vi "rethinkdb_json_type_cast.vi"(7 "type":variant, 8 "error in (no error)":errorcluster, 9 "allow missing? (F)":bool, 11 "json object":variant) -> (0 "error out":errorcluster, 1 "all keys found?":bool, 2 "data string":string, 3 "type string":i16[](array[numeric]))   [LabVIEW 2017]
uses:
  <vilib>/Utility/Data Type/Type Definitions/Data Type.ctl
  <vilib>/Utility/Data Type/NI_Data Type.lvlib
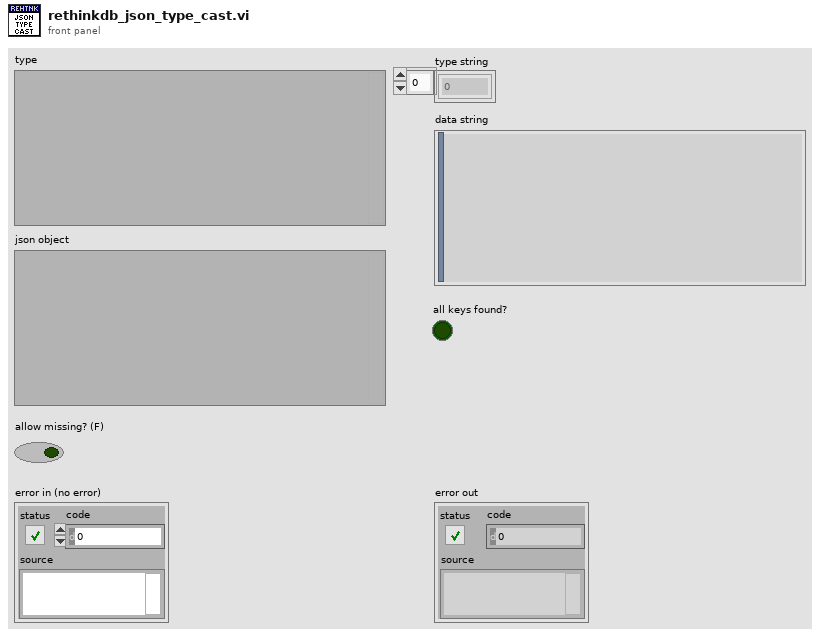
[diagram p1: front panel]
types:
  T1 = typedef "NI_Data Type.lvlib/Data Type.ctl" = enum8{"Invalid Type", "Void", "I8", "I16", "I32", "I64", "U8", "U16", "U32", "U64", "Single Float", "Double Float", "Extended Float", "Single Complex", "Double Complex", "Extended Complex", "Enum U8", "Enum U16", "Enum U32", "Enum U64", "Single Float With Unit", "Double Float With Unit", "Extended Float With Unit", "Single Complex with Unit", "Double Complex with Unit", "Extended Complex with Unit", "Boolean", "String", "Path", "Picture", "Tag", "Array", "Cluster", "Variant", "LV Variant", "Waveform", "Timestamp", "Digital Waveform", "Digital Data", "ExpressData", "Refnum", "External Data", "VI", "Poly VI", "LabVIEW Class Instance", "Fixed Point"}
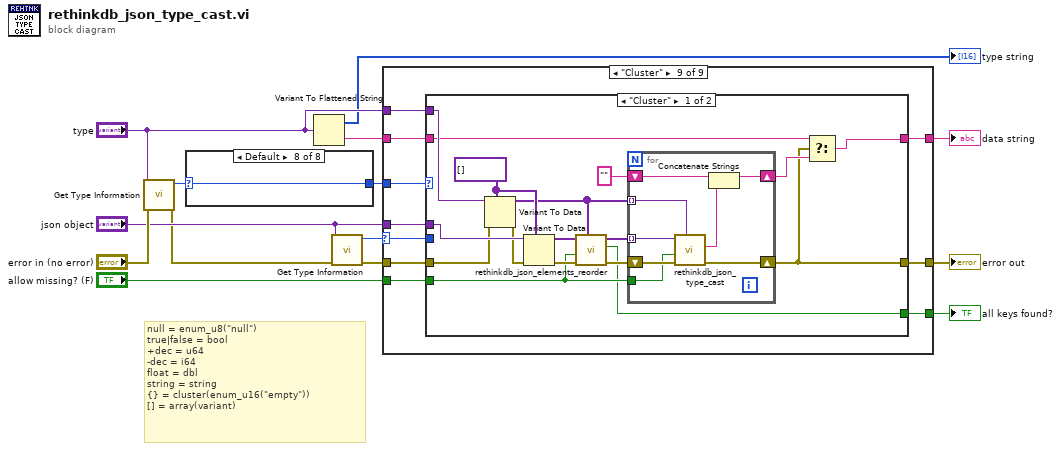
[diagram p0: block diagram]
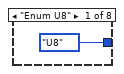
[diagram p2: hidden frame]
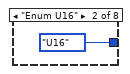
[diagram p3: hidden frame]
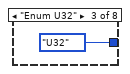
[diagram p4: hidden frame]
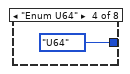
[diagram p5: hidden frame]
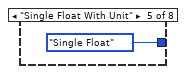
[diagram p6: hidden frame]
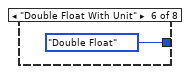
[diagram p7: hidden frame]
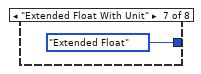
[diagram p8: hidden frame]
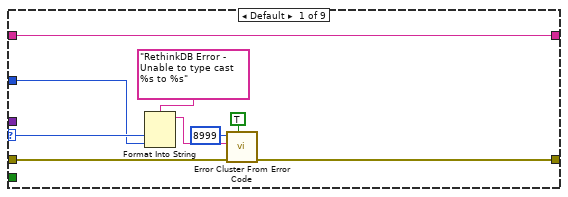
[diagram p9: hidden frame]
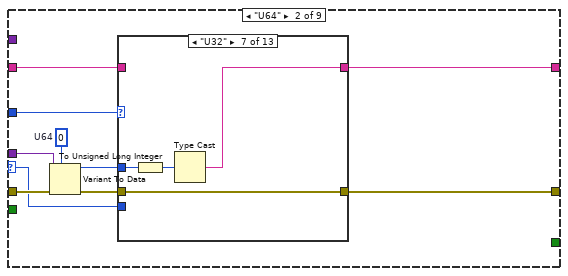
[diagram p10: hidden frame]
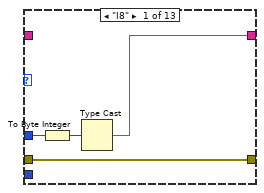
[diagram p11: hidden frame]
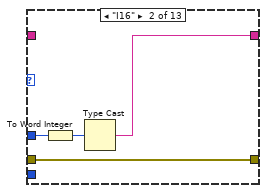
[diagram p12: hidden frame]
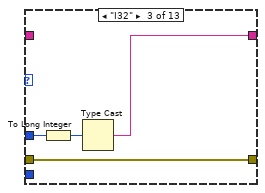
[diagram p13: hidden frame]
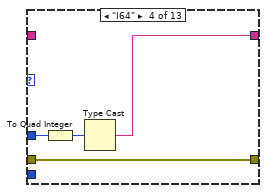
[diagram p14: hidden frame]
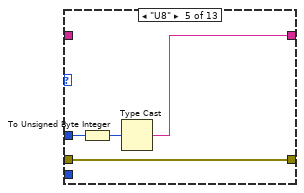
[diagram p15: hidden frame]
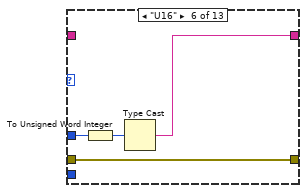
[diagram p16: hidden frame]
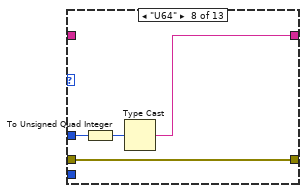
[diagram p17: hidden frame]
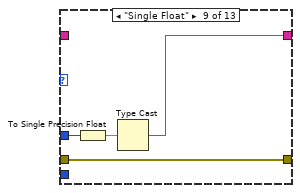
[diagram p18: hidden frame]
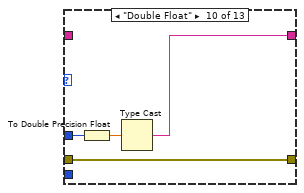
[diagram p19: hidden frame]
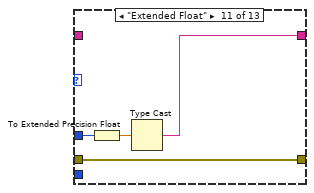
[diagram p20: hidden frame]
diagram:
  # "null = enum_u8(\"null\")\ntrue|false = bool\n+dec = u64\n-dec = i64\nfloat = dbl\nstring = string\n{} = cluster(enum_u16(\"empty\"))\n[] = array(variant)"
  n1 = call <vilib>:"Get Type Information.vi"("error in (no error)"="error in (no error)", "Variant"="type") -> ("error out"=w9:errorcluster, "Type"=w6:T1)  [unwired: 5 in, 3 out]
  n2 = case shown="Default" w6 {
    selector: w6 -> [_ _ _ _ _ _ _ w22]
    tunnel: [Data_Type."U8" ("Type") Data_Type."U16" ("Type") Data_Type."U32" ("Type") Data_Type."U64" ("Type") Data_Type."Single Float" ("Type") Data_Type."Double Float" ("Type") Data_Type."Extended Float" ("Type") w22] -> w5
    frame "Enum U8" {
    }
    frame "Enum U16" {
    }
    frame "Enum U32" {
    }
    frame "Enum U64" {
    }
    frame "Single Float With Unit" {
    }
    frame "Double Float With Unit" {
    }
    frame "Extended Float With Unit" {
    }
    frame Default {
    }
  }
  n3 = Variant To Flattened String(Variant="type") -> (data string=w4:string, 1:→"type string":i16[])
  n4 = call <vilib>:"Get Type Information.vi"("error in (no error)"=w9, "Variant"="json object") -> ("error out"=w7:errorcluster, "Type"=w8:T1)  [unwired: 5 in, 3 out]
  n5 = case shown="\"Cluster\"" w8 {
    selector: w8 -> [w25 w34 w102 w169 w235 w303 _ _ w368]
    tunnel: w7 -> [w31 w41 w108 w175 w243 w310 w332 w351 w367]
    tunnel: [w30 w35 w99 w166 w236 w304 w327 w346 w370] -> w12
    tunnel: w5 -> [w24 w37 w104 w171 w240 w307 w329 w348 w369]
    tunnel: "json object" -> [_ w40 w107 w174 w242 w309 w331 w350 w366]
    tunnel: w4 -> [w23 w33 w101 w168 w234 w302 w325 w344 w364]
    tunnel: [w23 w32 w100 w167 w233 w301 w324 w344 w365] -> w10
    tunnel: "type" -> [_ _ _ _ _ _ _ _ w363]
    tunnel: "allow missing? (F)" -> [_ _ _ _ _ _ _ _ w362]
    tunnel: [_ _ _ _ _ _ _ _ w361] -> w1
    frame Default {
      n6 = Format Into String(format string="RethinkDB Error - Unable to type cast %s to %s" ("error message (\"\")"), w25, w24) -> (resulting string=w26:string)  [unwired: 2 in, 1 out]
      n7 = call <vilib>:"Error Cluster From Error Code.vi"("show call chain? (False)"=TRUE, "error in (no error)"=w31, "error message (\"\")"=w26, "error code (0)"=8999) -> ("error out"=w30:errorcluster)  [unwired: 5 in]
    }
    frame "U64" {
      w39 = u64 0  # U64
      n8 = Variant To Data(error in=w41, type=w39, Variant=w40) -> (data=w36:u64, error out=w38:errorcluster)
      n9 = case shown="\"U32\"" w37 {
        selector: w37 -> [_ _ _ _ _ _ _ _ _ _ _ _ w91]
        tunnel: [w45 w49 w53 w57 w61 w65 w69 w73 w77 w81 w85 w89 w92] -> w35
        tunnel: w38 -> [w45 w49 w53 w57 w61 w65 w69 w73 w77 w81 w85 w89 w93]
        tunnel: w36 -> [w44 w48 w52 w56 w60 w64 w68 w72 w76 w80 w84 w87 _]
        tunnel: [w42 w46 w50 w54 w58 w62 w66 w70 w74 w78 w82 w88 w98] -> w32
        tunnel: w33 -> [_ _ _ _ _ _ _ _ _ _ _ _ w98]
        tunnel: w34 -> [_ _ _ _ _ _ _ _ _ _ _ _ w90]
        frame "I8" {
          n10 = To Byte Integer(number=w44) -> (8bit integer=w43:i8)
          n11 = Type Cast(x=w43) -> (*(type *) &x=w42:string)  [unwired: 1 in]
        }
        frame "I16" {
          n12 = To Word Integer(number=w48) -> (16bit integer=w47:i16)
          n13 = Type Cast(x=w47) -> (*(type *) &x=w46:string)  [unwired: 1 in]
        }
        frame "I32" {
          n14 = To Long Integer(number=w52) -> (32bit integer=w51:i32)
          n15 = Type Cast(x=w51) -> (*(type *) &x=w50:string)  [unwired: 1 in]
        }
        frame "I64" {
          n16 = To Quad Integer(1:w56) -> (0:w55:i64)
          n17 = Type Cast(x=w55) -> (*(type *) &x=w54:string)  [unwired: 1 in]
        }
        frame "U8" {
          n18 = To Unsigned Byte Integer(number=w60) -> (unsigned 8bit integer=w59:u8)
          n19 = Type Cast(x=w59) -> (*(type *) &x=w58:string)  [unwired: 1 in]
        }
        frame "U16" {
          n20 = To Unsigned Word Integer(number=w64) -> (unsigned 16bit integer=w63:u16)
          n21 = Type Cast(x=w63) -> (*(type *) &x=w62:string)  [unwired: 1 in]
        }
        frame "U32" {
          n22 = To Unsigned Long Integer(number=w68) -> (unsigned 32bit integer=w67:u32)
          n23 = Type Cast(x=w67) -> (*(type *) &x=w66:string)  [unwired: 1 in]
        }
        frame "U64" {
          n24 = To Unsigned Quad Integer(1:w72) -> (0:w71:u64)
          n25 = Type Cast(x=w71) -> (*(type *) &x=w70:string)  [unwired: 1 in]
        }
        frame "Single Float" {
          n26 = To Single Precision Float(number=w76) -> (single precision float=w75:sgl)
          n27 = Type Cast(x=w75) -> (*(type *) &x=w74:string)  [unwired: 1 in]
        }
        frame "Double Float" {
          n28 = To Double Precision Float(number=w80) -> (double precision float=w79:dbl)
          n29 = Type Cast(x=w79) -> (*(type *) &x=w78:string)  [unwired: 1 in]
        }
        frame "Extended Float" {
          n30 = To Extended Precision Float(1:w84) -> (0:w83:ext)
          n31 = Type Cast(x=w83) -> (*(type *) &x=w82:string)  [unwired: 1 in]
        }
        frame "Boolean" {
          n32 = Not Equal To 0?(x=w87) -> (x != 0?=w86:bool)
          n33 = Type Cast(x=w86) -> (*(type *) &x=w88:string)  [unwired: 1 in]
        }
        frame Default {
          n34 = Format Into String(format string="RethinkDB Error - Unable to type cast %s to %s" ("error message (\"\")"), w90, w91) -> (resulting string=w94:string)  [unwired: 2 in, 1 out]
          n35 = call <vilib>:"Error Cluster From Error Code.vi"("show call chain? (False)"=TRUE, "error in (no error)"=w93, "error message (\"\")"=w94, "error code (0)"=8999) -> ("error out"=w92:errorcluster)  [unwired: 5 in]
        }
      }
    }
    frame "I64" {
      w106 = i64 0  # I64
      n36 = Variant To Data(error in=w108, type=w106, Variant=w107) -> (data=w103:i64, error out=w105:errorcluster)
      n37 = case shown="Default" w104 {
        selector: w104 -> [_ _ _ _ _ _ _ _ _ _ _ _ w158]
        tunnel: [w112 w116 w120 w124 w128 w132 w136 w140 w144 w148 w152 w156 w159] -> w99
        tunnel: w105 -> [w112 w116 w120 w124 w128 w132 w136 w140 w144 w148 w152 w156 w160]
        tunnel: w103 -> [w111 w115 w119 w123 w127 w131 w135 w139 w143 w147 w151 w154 _]
        tunnel: [w109 w113 w117 w121 w125 w129 w133 w137 w141 w145 w149 w155 w165] -> w100
        tunnel: w101 -> [_ _ _ _ _ _ _ _ _ _ _ _ w165]
        tunnel: w102 -> [_ _ _ _ _ _ _ _ _ _ _ _ w157]
        frame "I8" {
          n38 = To Byte Integer(number=w111) -> (8bit integer=w110:i8)
          n39 = Type Cast(x=w110) -> (*(type *) &x=w109:string)  [unwired: 1 in]
        }
        frame "I16" {
          n40 = To Word Integer(number=w115) -> (16bit integer=w114:i16)
          n41 = Type Cast(x=w114) -> (*(type *) &x=w113:string)  [unwired: 1 in]
        }
        frame "I32" {
          n42 = To Long Integer(number=w119) -> (32bit integer=w118:i32)
          n43 = Type Cast(x=w118) -> (*(type *) &x=w117:string)  [unwired: 1 in]
        }
        frame "I64" {
          n44 = To Quad Integer(1:w123) -> (0:w122:i64)
          n45 = Type Cast(x=w122) -> (*(type *) &x=w121:string)  [unwired: 1 in]
        }
        frame "U8" {
          n46 = To Unsigned Byte Integer(number=w127) -> (unsigned 8bit integer=w126:u8)
          n47 = Type Cast(x=w126) -> (*(type *) &x=w125:string)  [unwired: 1 in]
        }
        frame "U16" {
          n48 = To Unsigned Word Integer(number=w131) -> (unsigned 16bit integer=w130:u16)
          n49 = Type Cast(x=w130) -> (*(type *) &x=w129:string)  [unwired: 1 in]
        }
        frame "U32" {
          n50 = To Unsigned Long Integer(number=w135) -> (unsigned 32bit integer=w134:u32)
          n51 = Type Cast(x=w134) -> (*(type *) &x=w133:string)  [unwired: 1 in]
        }
        frame "U64" {
          n52 = To Unsigned Quad Integer(1:w139) -> (0:w138:u64)
          n53 = Type Cast(x=w138) -> (*(type *) &x=w137:string)  [unwired: 1 in]
        }
        frame "Single Float" {
          n54 = To Single Precision Float(number=w143) -> (single precision float=w142:sgl)
          n55 = Type Cast(x=w142) -> (*(type *) &x=w141:string)  [unwired: 1 in]
        }
        frame "Double Float" {
          n56 = To Double Precision Float(number=w147) -> (double precision float=w146:dbl)
          n57 = Type Cast(x=w146) -> (*(type *) &x=w145:string)  [unwired: 1 in]
        }
        frame "Extended Float" {
          n58 = To Extended Precision Float(1:w151) -> (0:w150:ext)
          n59 = Type Cast(x=w150) -> (*(type *) &x=w149:string)  [unwired: 1 in]
        }
        frame "Boolean" {
          n60 = Not Equal To 0?(x=w154) -> (x != 0?=w153:bool)
          n61 = Type Cast(x=w153) -> (*(type *) &x=w155:string)  [unwired: 1 in]
        }
        frame Default {
          n62 = Format Into String(format string="RethinkDB Error - Unable to type cast %s to %s" ("error message (\"\")"), w157, w158) -> (resulting string=w161:string)  [unwired: 2 in, 1 out]
          n63 = call <vilib>:"Error Cluster From Error Code.vi"("show call chain? (False)"=TRUE, "error in (no error)"=w160, "error message (\"\")"=w161, "error code (0)"=8999) -> ("error out"=w159:errorcluster)  [unwired: 5 in]
        }
      }
    }
    frame "Double Float" {
      w173 = 0.0  # DBL
      n64 = Variant To Data(error in=w175, type=w173, Variant=w174) -> (data=w170:dbl, error out=w172:errorcluster)
      n65 = case shown="Default" w171 {
        selector: w171 -> [_ _ _ _ _ _ _ _ _ _ _ _ w225]
        tunnel: [w179 w183 w187 w191 w195 w199 w203 w207 w211 w215 w219 w223 w226] -> w166
        tunnel: w172 -> [w179 w183 w187 w191 w195 w199 w203 w207 w211 w215 w219 w223 w227]
        tunnel: w170 -> [w178 w182 w186 w190 w194 w198 w202 w206 w210 w214 w218 w221 _]
        tunnel: [w176 w180 w184 w188 w192 w196 w200 w204 w208 w212 w216 w222 w232] -> w167
        tunnel: w168 -> [_ _ _ _ _ _ _ _ _ _ _ _ w232]
        tunnel: w169 -> [_ _ _ _ _ _ _ _ _ _ _ _ w224]
        frame "I8" {
          n66 = To Byte Integer(number=w178) -> (8bit integer=w177:i8)
          n67 = Type Cast(x=w177) -> (*(type *) &x=w176:string)  [unwired: 1 in]
        }
        frame "I16" {
          n68 = To Word Integer(number=w182) -> (16bit integer=w181:i16)
          n69 = Type Cast(x=w181) -> (*(type *) &x=w180:string)  [unwired: 1 in]
        }
        frame "I32" {
          n70 = To Long Integer(number=w186) -> (32bit integer=w185:i32)
          n71 = Type Cast(x=w185) -> (*(type *) &x=w184:string)  [unwired: 1 in]
        }
        frame "I64" {
          n72 = To Quad Integer(1:w190) -> (0:w189:i64)
          n73 = Type Cast(x=w189) -> (*(type *) &x=w188:string)  [unwired: 1 in]
        }
        frame "U8" {
          n74 = To Unsigned Byte Integer(number=w194) -> (unsigned 8bit integer=w193:u8)
          n75 = Type Cast(x=w193) -> (*(type *) &x=w192:string)  [unwired: 1 in]
        }
        frame "U16" {
          n76 = To Unsigned Word Integer(number=w198) -> (unsigned 16bit integer=w197:u16)
          n77 = Type Cast(x=w197) -> (*(type *) &x=w196:string)  [unwired: 1 in]
        }
        frame "U32" {
          n78 = To Unsigned Long Integer(number=w202) -> (unsigned 32bit integer=w201:u32)
          n79 = Type Cast(x=w201) -> (*(type *) &x=w200:string)  [unwired: 1 in]
        }
        frame "U64" {
          n80 = To Unsigned Quad Integer(1:w206) -> (0:w205:u64)
          n81 = Type Cast(x=w205) -> (*(type *) &x=w204:string)  [unwired: 1 in]
        }
        frame "Single Float" {
          n82 = To Single Precision Float(number=w210) -> (single precision float=w209:sgl)
          n83 = Type Cast(x=w209) -> (*(type *) &x=w208:string)  [unwired: 1 in]
        }
        frame "Double Float" {
          n84 = To Double Precision Float(number=w214) -> (double precision float=w213:dbl)
          n85 = Type Cast(x=w213) -> (*(type *) &x=w212:string)  [unwired: 1 in]
        }
        frame "Extended Float" {
          n86 = To Extended Precision Float(1:w218) -> (0:w217:ext)
          n87 = Type Cast(x=w217) -> (*(type *) &x=w216:string)  [unwired: 1 in]
        }
        frame "Boolean" {
          n88 = Not Equal To 0?(x=w221) -> (x != 0?=w220:bool)
          n89 = Type Cast(x=w220) -> (*(type *) &x=w222:string)  [unwired: 1 in]
        }
        frame Default {
          n90 = Format Into String(format string="RethinkDB Error - Unable to type cast %s to %s" ("error message (\"\")"), w224, w225) -> (resulting string=w228:string)  [unwired: 2 in, 1 out]
          n91 = call <vilib>:"Error Cluster From Error Code.vi"("show call chain? (False)"=TRUE, "error in (no error)"=w227, "error message (\"\")"=w228, "error code (0)"=8999) -> ("error out"=w226:errorcluster)  [unwired: 5 in]
        }
      }
    }
    frame "Boolean" {
      n92 = Variant To Data(error in=w243, type=FALSE, Variant=w242) -> (data=w239:bool, error out=w241:errorcluster)
      n93 = Boolean To (0,1)(Boolean=w239) -> (0, 1=w237:i16)
      n94 = case shown="Default" w240 {
        selector: w240 -> [_ _ _ _ _ _ _ _ _ _ _ _ w293]
        tunnel: [w247 w251 w255 w259 w263 w267 w271 w275 w279 w283 w287 w291 w294] -> w236
        tunnel: w241 -> [w247 w251 w255 w259 w263 w267 w271 w275 w279 w283 w287 w291 w295]
        tunnel: w237 -> [w246 w250 w254 w258 w262 w266 w270 w274 w278 w282 w286 w289 _]
        tunnel: [w244 w248 w252 w256 w260 w264 w268 w272 w276 w280 w284 w290 w300] -> w233
        tunnel: w234 -> [_ _ _ _ _ _ _ _ _ _ _ _ w300]
        tunnel: w235 -> [_ _ _ _ _ _ _ _ _ _ _ _ w292]
        frame "I8" {
          n95 = To Byte Integer(number=w246) -> (8bit integer=w245:i8)
          n96 = Type Cast(x=w245) -> (*(type *) &x=w244:string)  [unwired: 1 in]
        }
        frame "I16" {
          n97 = To Word Integer(number=w250) -> (16bit integer=w249:i16)
          n98 = Type Cast(x=w249) -> (*(type *) &x=w248:string)  [unwired: 1 in]
        }
        frame "I32" {
          n99 = To Long Integer(number=w254) -> (32bit integer=w253:i32)
          n100 = Type Cast(x=w253) -> (*(type *) &x=w252:string)  [unwired: 1 in]
        }
        frame "I64" {
          n101 = To Quad Integer(1:w258) -> (0:w257:i64)
          n102 = Type Cast(x=w257) -> (*(type *) &x=w256:string)  [unwired: 1 in]
        }
        frame "U8" {
          n103 = To Unsigned Byte Integer(number=w262) -> (unsigned 8bit integer=w261:u8)
          n104 = Type Cast(x=w261) -> (*(type *) &x=w260:string)  [unwired: 1 in]
        }
        frame "U16" {
          n105 = To Unsigned Word Integer(number=w266) -> (unsigned 16bit integer=w265:u16)
          n106 = Type Cast(x=w265) -> (*(type *) &x=w264:string)  [unwired: 1 in]
        }
        frame "U32" {
          n107 = To Unsigned Long Integer(number=w270) -> (unsigned 32bit integer=w269:u32)
          n108 = Type Cast(x=w269) -> (*(type *) &x=w268:string)  [unwired: 1 in]
        }
        frame "U64" {
          n109 = To Unsigned Quad Integer(1:w274) -> (0:w273:u64)
          n110 = Type Cast(x=w273) -> (*(type *) &x=w272:string)  [unwired: 1 in]
        }
        frame "Single Float" {
          n111 = To Single Precision Float(number=w278) -> (single precision float=w277:sgl)
          n112 = Type Cast(x=w277) -> (*(type *) &x=w276:string)  [unwired: 1 in]
        }
        frame "Double Float" {
          n113 = To Double Precision Float(number=w282) -> (double precision float=w281:dbl)
          n114 = Type Cast(x=w281) -> (*(type *) &x=w280:string)  [unwired: 1 in]
        }
        frame "Extended Float" {
          n115 = To Extended Precision Float(1:w286) -> (0:w285:ext)
          n116 = Type Cast(x=w285) -> (*(type *) &x=w284:string)  [unwired: 1 in]
        }
        frame "Boolean" {
          n117 = Not Equal To 0?(x=w289) -> (x != 0?=w288:bool)
          n118 = Type Cast(x=w288) -> (*(type *) &x=w290:string)  [unwired: 1 in]
        }
        frame Default {
          n119 = Format Into String(format string="RethinkDB Error - Unable to type cast %s to %s" ("error message (\"\")"), w292, w293) -> (resulting string=w296:string)  [unwired: 2 in, 1 out]
          n120 = call <vilib>:"Error Cluster From Error Code.vi"("show call chain? (False)"=TRUE, "error in (no error)"=w295, "error message (\"\")"=w296, "error code (0)"=8999) -> ("error out"=w294:errorcluster)  [unwired: 5 in]
        }
      }
    }
    frame "String" {
      n121 = Variant To Data(error in=w310, type="", Variant=w309) -> (data=w305:string, error out=w308:errorcluster)
      n122 = case shown="Default" w307 {
        selector: w307 -> [_ w316]
        tunnel: [w314 w317] -> w304
        tunnel: w308 -> [w314 w318]
        tunnel: w305 -> [w313 _]
        tunnel: [w312 w323] -> w301
        tunnel: w302 -> [_ w323]
        tunnel: w303 -> [_ w315]
        frame "String" {
          n123 = To Variant(anything=w313) -> (Variant=w311:variant)
          n124 = Variant To Flattened String(Variant=w311) -> (data string=w312:string)  [unwired: 1 out]
        }
        frame Default {
          n125 = Format Into String(format string="RethinkDB Error - Unable to type cast %s to %s" ("error message (\"\")"), w315, w316) -> (resulting string=w319:string)  [unwired: 2 in, 1 out]
          n126 = call <vilib>:"Error Cluster From Error Code.vi"("show call chain? (False)"=TRUE, "error in (no error)"=w318, "error message (\"\")"=w319, "error code (0)"=8999) -> ("error out"=w317:errorcluster)  [unwired: 5 in]
        }
      }
    }
    frame "Enum U8" {
      w328 = enum8{"null"}."null"  # null
      n127 = Variant To Data(error in=w332, type=w328, Variant=w331) -> (data=w326:enum8{"null"}, error out=w330:errorcluster)
      n128 = case shown="Default" w329 {
        selector: w329 -> [_ w336]
        tunnel: [w334 w337] -> w327
        tunnel: w330 -> [w334 w338]
        tunnel: [w333 w343] -> w324
        tunnel: w325 -> [w333 w343]
        tunnel: w326 -> [_ w335]
        frame "I8".."Extended Float", "Boolean", "String" {
          # "use default"
        }
        frame Default {
          n129 = Format Into String(format string="RethinkDB Error - Unable to type cast %s to %s" ("error message (\"\")"), w335, w336) -> (resulting string=w339:string)  [unwired: 2 in, 1 out]
          n130 = call <vilib>:"Error Cluster From Error Code.vi"("show call chain? (False)"=TRUE, "error in (no error)"=w338, "error message (\"\")"=w339, "error code (0)"=8999) -> ("error out"=w337:errorcluster)  [unwired: 5 in]
        }
      }
    }
    frame "Enum U16" {
      w347 = enum16{"empty"}."empty"  # empty
      n131 = Variant To Data(error in=w351, type=w347, Variant=w350) -> (data=w345:enum16{"empty"}, error out=w349:errorcluster)
      n132 = case shown="Default" w348 {
        selector: w348 -> [_ w354]
        tunnel: [w352 w355] -> w346
        tunnel: w349 -> [w352 w356]
        tunnel: w345 -> [_ w353]
        frame "I8".."Extended Float", "Boolean", "String" {
          # "use default"
        }
        frame Default {
          n133 = Format Into String(format string="RethinkDB Error - Unable to type cast %s to %s" ("error message (\"\")"), w353, w354) -> (resulting string=w357:string)  [unwired: 2 in, 1 out]
          n134 = call <vilib>:"Error Cluster From Error Code.vi"("show call chain? (False)"=TRUE, "error in (no error)"=w356, "error message (\"\")"=w357, "error code (0)"=8999) -> ("error out"=w355:errorcluster)  [unwired: 5 in]
        }
      }
    }
    frame "Cluster" {
      n135 = case shown="\"Cluster\"" w369 {
        selector: w369 -> [_ w398]
        tunnel: [w383 w399] -> w370
        tunnel: w367 -> [w377 w400]
        tunnel: w368 -> [_ w397]
        tunnel: w366 -> [w387 _]
        tunnel: w363 -> [w386 _]
        tunnel: [w381 w396] -> w365
        tunnel: w364 -> [w382 w396]
        tunnel: w362 -> [w372 _]
        tunnel: [w371 _] -> w361
        frame "Cluster" {
          w375 = variant[] []
          n136 = Variant To Data(error in=w377, type=w375, Variant=w386) -> (data=w374:variant[], error out=w376:errorcluster)
          n137 = Variant To Data(error in=w376, type=w375, Variant=w387) -> (data=w379:variant[], error out=w378:errorcluster)
          n138 = call "rethinkdb_json_elements_reorder.vi"("type elements"=w374, "error in (no error)"=w378, "allow missing?"=w372, "json elements"=w379) -> ("error out"=w380:errorcluster, "all keys found?"=w371:bool, "reordered json elements"=w373:variant[])  [unwired: 5 in]
          n139 = for {
            tunnel: w373 -> [w389] mode=indexing
            shift-right: [w394] -> w383
            shift-left: w380 -> [w395]
            tunnel: w374 -> [w393] mode=indexing
            shift-right: [w391] -> w384
            shift-left: "" -> [w392]
            tunnel: w372 -> [w388]
            n140 = call "rethinkdb_json_type_cast.vi"("type"=w393, "error in (no error)"=w395, "allow missing? (F)"=w388, "json object"=w389) -> ("error out"=w394:errorcluster, "data string"=w390:string)  [unwired: 4 in, 2 out]
            n141 = Concatenate Strings(w392, w390) -> (w391:string)
          }
          n142 = Select(t=w382, s=w383, f=w384) -> (s? t:f=w381:string)
        }
        frame Default {
          n143 = Format Into String(format string="RethinkDB Error - Unable to type cast %s to %s" ("error message (\"\")"), w397, w398) -> (resulting string=w401:string)  [unwired: 2 in, 1 out]
          n144 = call <vilib>:"Error Cluster From Error Code.vi"("show call chain? (False)"=TRUE, "error in (no error)"=w400, "error message (\"\")"=w401, "error code (0)"=8999) -> ("error out"=w399:errorcluster)  [unwired: 5 in]
        }
      }
    }
  }
  "error out" <- w12
  "all keys found?" <- w1
  "data string" <- w10
